vi "ParseDeviceData.vi"(8 "error in (no error)":errorcluster, 10 "Packet0":u8[](array[numeric])) -> (0 "error out":errorcluster, 2 "DataGood?":bool, 3 "Cluster":T1 {"DevInfo"."ASICtrim" format="%02x"})   [LabVIEW 2015]
uses:
  Controls/DeviceInfo.ctl
  Controls/InfoPacket.ctl
  Controls/Gen2 FT Globals.vi
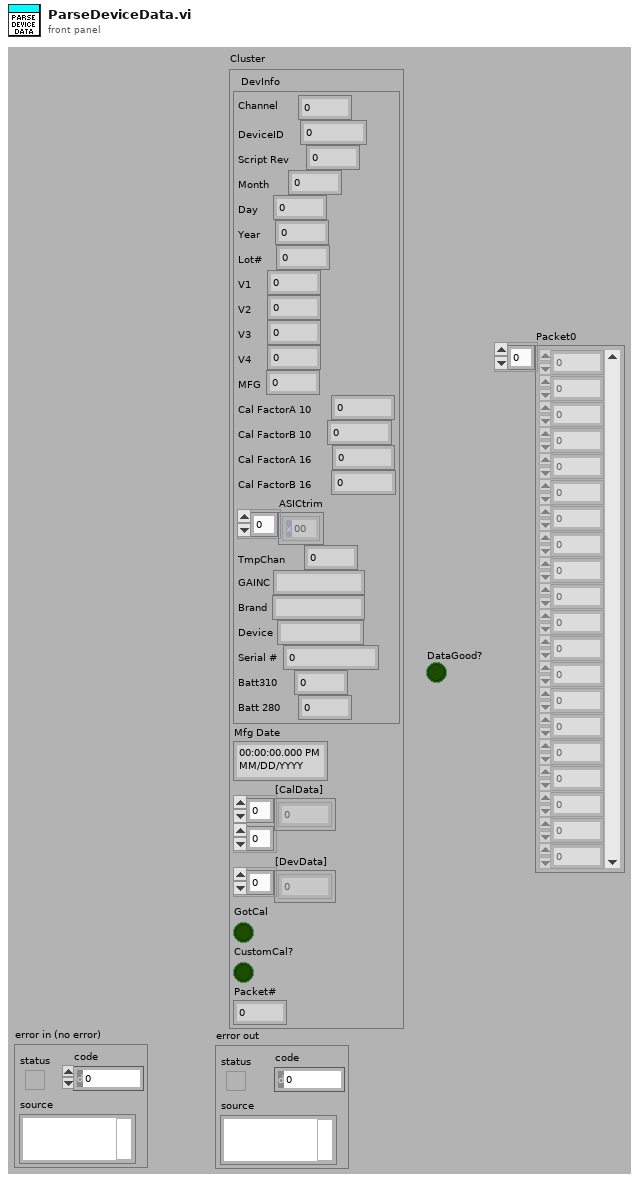
[diagram p1: front panel]
types:
  T1 = typedef "DeviceInfo.ctl" = cluster{"DevInfo":T2, "Mfg Date":timestamp, "[CalData]":u8[][], "[DevData]":u8[], "GotCal":bool, "CustomCal?":bool, "Packet#":i32}
  T2 = typedef "InfoPacket.ctl" = cluster{"Channel":u8, "DeviceID":u32, "Script Rev":u8, "Month":u8, "Day":u8, "Year":u8, "Lot#":u32, "V1":u16, "V2":u16, "V3":u16, "V4":u16, "MFG":u8, "Cal FactorA 10":u8, "Cal FactorB 10  ":u8, "Cal FactorA 16":u8, "Cal FactorB 16":u8, "ASICtrim":u8[], "TmpChan":u8, "GAINC":string, "Brand":string, "Device":string, "Serial #":u64, "Batt310":u16, "Batt 280":u16}
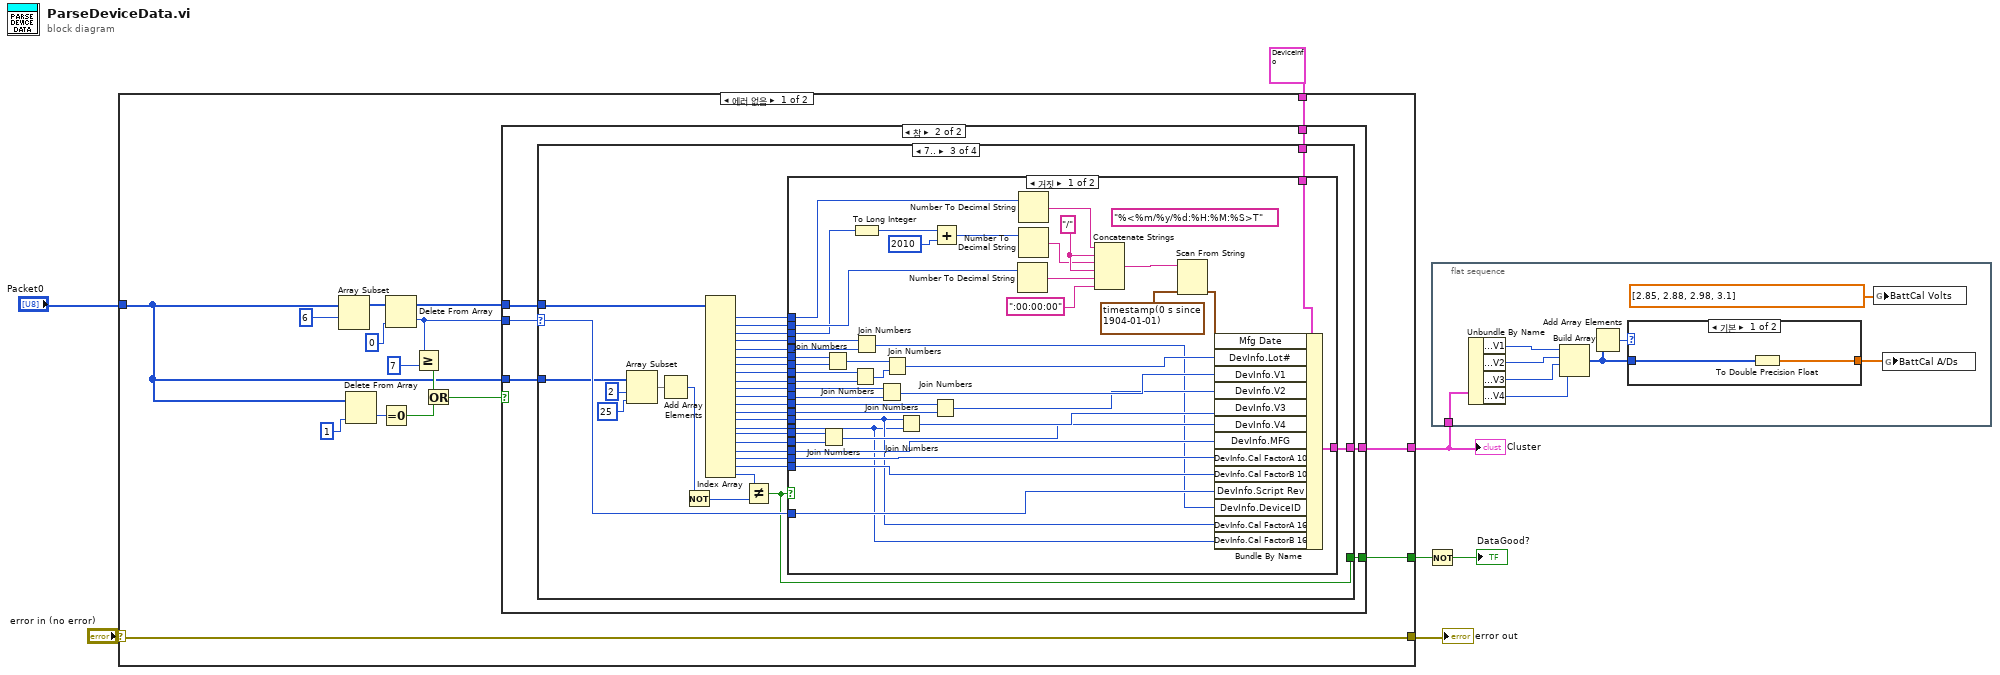
[diagram p0: block diagram]
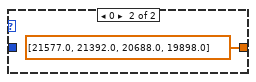
[diagram p2: hidden frame]
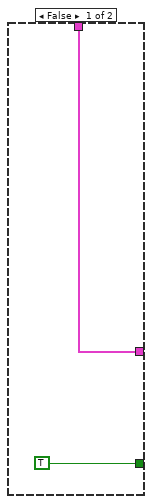
[diagram p3: hidden frame]
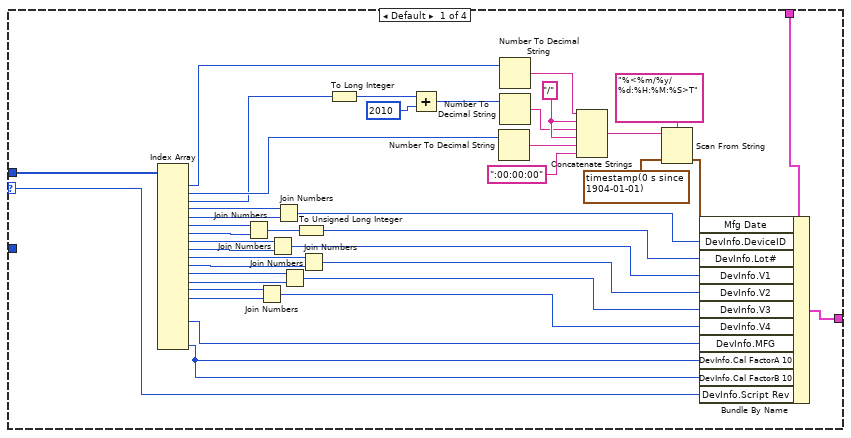
[diagram p4: hidden frame]
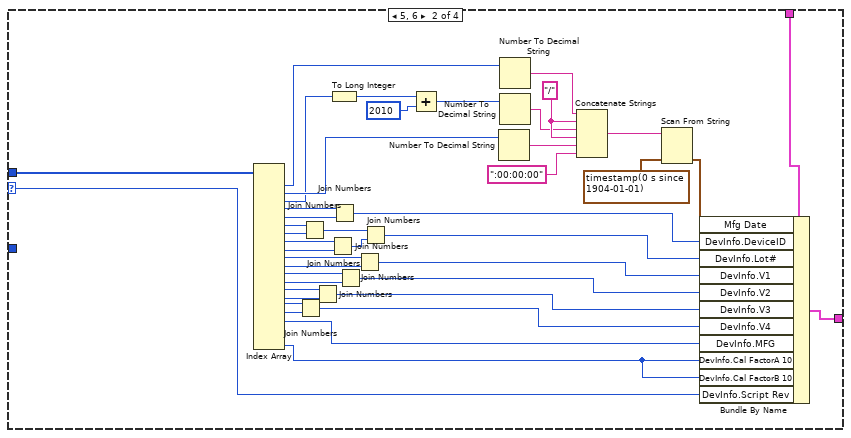
[diagram p5: hidden frame]
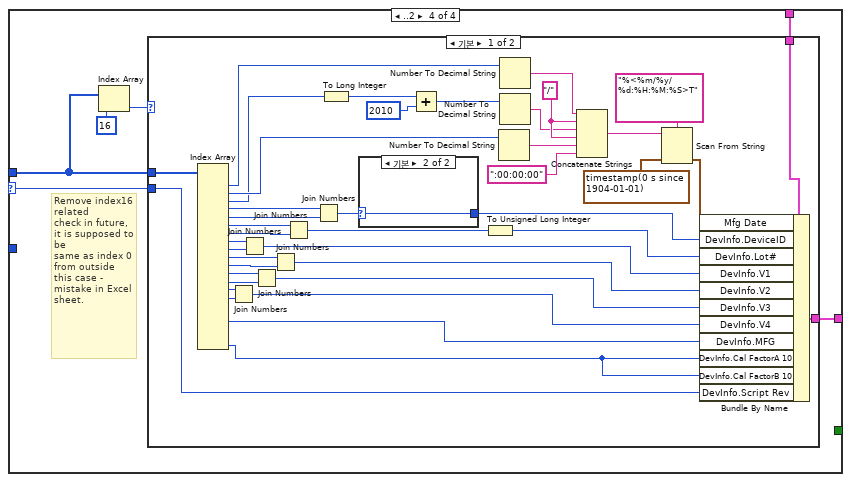
[diagram p7: hidden frame]
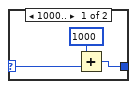
[diagram p8: hidden frame]
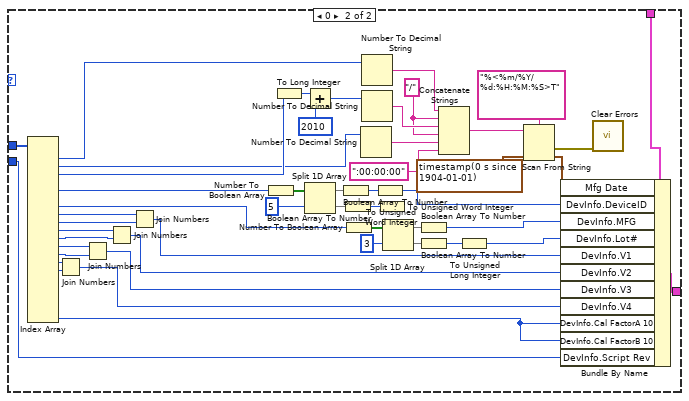
[diagram p9: hidden frame]
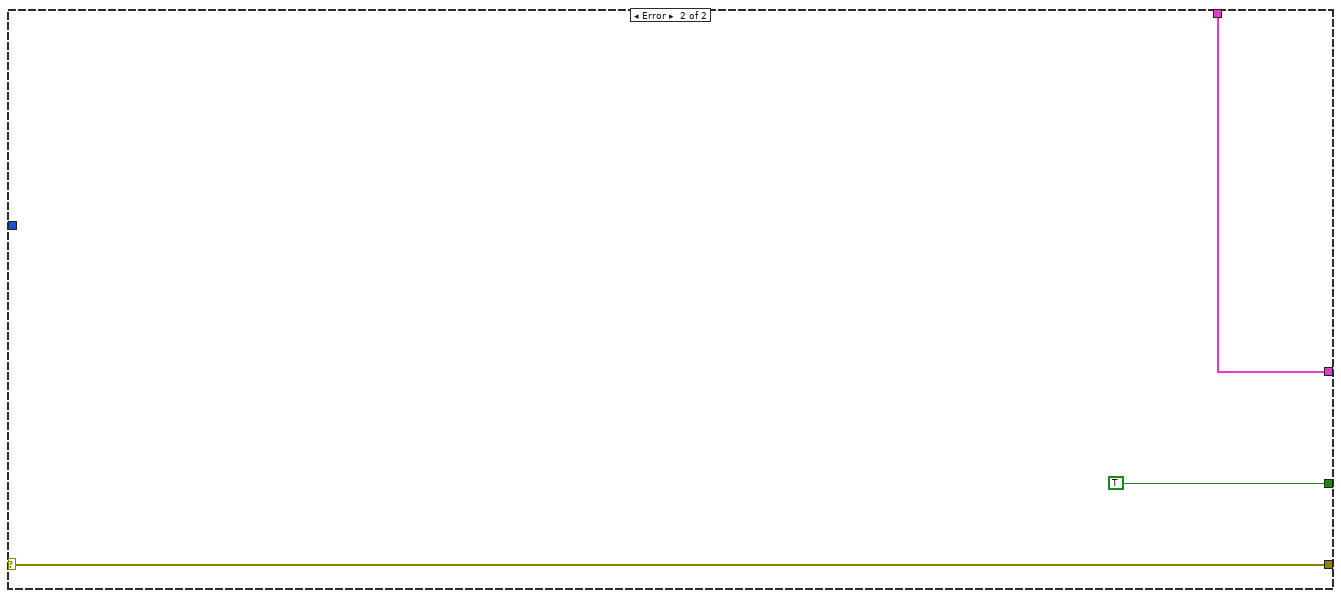
[diagram p10: hidden frame]
diagram:
  n1 = case shown="에러 없음" "error in (no error)" {
    selector: "error in (no error)" -> [w23 w291]
    tunnel: [w23 w291] -> w6
    tunnel: T1 {"DevInfo"={"Channel"=0, "DeviceID"=0, "Script Rev"=0, "Month"=0, "Day"=0, "Year"=0, "Lot#"=0, "V1"=0, "V2"=0, "V3"=0, "V4"=0, "MFG"=0, "Cal FactorA 10"=0, "Cal FactorB 10  "=0, "Cal FactorA 16"=0, "Cal FactorB 16"=0, "ASICtrim"=[], "TmpChan"=0, "GAINC"="", "Brand"="", "Device"="", "Serial #"=0, "Batt310"=0, "Batt 280"=0}, "Mfg Date"=timestamp(0 s since 1904-01-01), "[CalData]"=[], "[DevData]"=[], "GotCal"=FALSE, "CustomCal?"=FALSE, "Packet#"=0} -> [w22 w290]
    tunnel: [w21 w290] -> w3
    tunnel: "Packet0" -> [w8 _]
    tunnel: [w16 TRUE] -> w2
    frame No Error {
      n2 = Array Subset(array=w8, index=6) -> (w20:u8[])  [unwired: 1 in]
      n3 = Delete From Array(array=w8, index=1) -> (deleted portion=w14:u8)  [unwired: 1 in, 1 out]
      n4 = Equal To 0?(x=w14) -> (x = 0?=w9:bool)
      n5 = Delete From Array(array=w20, index=0) -> (deleted portion=w13:u8, array with subset deleted=w17:u8[])  [unwired: 1 in]
      n6 = Greater Or Equal?(x=w13, y=u8 7) -> (x >= y?=w10:bool)
      n7 = Or(x=w10, y=w9) -> (x .or. y?=w11:bool)
      n8 = case shown="참" w11 {
        tunnel: w22 -> [w25 w31]
        tunnel: [w25 w30] -> w21
        tunnel: w17 -> [_ w29]
        tunnel: w13 -> [_ w28]
        tunnel: [TRUE w27] -> w16
        tunnel: w8 -> [_ w26]
        frame False {
        }
        frame True {
          n9 = case shown="7.." w28 {
            selector: w28 -> [w68 w110 w143 w192]
            tunnel: w31 -> [w70 w112 w145 w194]
            tunnel: [w69 w111 w144 w193] -> w30
            tunnel: w29 -> [w71 w113 w122 w190]
            tunnel: w26 -> [_ _ w121 _]
            tunnel: [_ _ w114 _] -> w27
            frame Default {
              w58 = "/" ("string")
              n10 = Index Array(array=w71) -> (element #1=w63:u8, element #2=w64:u8, element #3=w52:u8, element #4=w66:u8, element #5=w67:u8, element #6=w50:u8, element #7=w51:u8, element #8=w47:u8, element #9=w46:u8, element #10=w45:u8, element #11=w44:u8, element #12=w43:u8, element #13=w42:u8, element #14=w41:u8, element #15=w40:u8, element #18=w38:u8, element #21=w32:u8)  [unwired: 21 in, 4 out]
              n11 = Join Numbers(hi=w50, lo=w51) -> ((hi.lo)=w39:u16)
              n12 = Join Numbers(hi=w41, lo=w40) -> ((hi.lo)=w33:u16)
              n13 = Join Numbers(hi=w47, lo=w46) -> ((hi.lo)=w36:u16)
              n14 = Join Numbers(hi=w66, lo=w67) -> ((hi.lo)=w48:u16)
              n15 = Join Numbers(hi=w43, lo=w42) -> ((hi.lo)=w34:u16)
              n16 = To Unsigned Long Integer(number=w39) -> (unsigned 32bit integer=w37:u32)
              n17 = Join Numbers(hi=w45, lo=w44) -> ((hi.lo)=w35:u16)
              n18 = To Long Integer(number=w52) -> (32bit integer=w54:i32)
              n19 = Add(x=w54, y=2010) -> (x+y=w65:i32)
              n20 = Number To Decimal String(number=w64) -> (decimal integer string=w59:string)  [unwired: 1 in]
              n21 = Number To Decimal String(number=w63) -> (decimal integer string=w56:string)  [unwired: 1 in]
              n22 = Number To Decimal String(number=w65) -> (decimal integer string=w57:string)  [unwired: 1 in]
              n23 = Concatenate Strings(w56, w58, w57, w58, w59, ":00:00:00" ("string")) -> (w62:string)
              n24 = Scan From String(format string="%<%m/%y/%d:%H:%M:%S>T", input string=w62, default 1=timestamp(0 s since 1904-01-01) ("current time")) -> (output 1=w49:timestamp)  [unwired: 2 in, 3 out]
              n25 = Bundle By Name(cluster=w70, "Mfg Date"=w49, "DevInfo.DeviceID"=w48, "DevInfo.Lot#"=w37, "DevInfo.V1"=w36, "DevInfo.V2"=w35, "DevInfo.V3"=w34, "DevInfo.V4"=w33, "DevInfo.MFG"=w38, "DevInfo.Cal FactorA 10"=w32, "DevInfo.Cal FactorB 10"=w32, "DevInfo.Script Rev"=w68) -> (w69:T1)
            }
            frame 5, 6 {
              w100 = "/" ("string")
              n26 = Index Array(array=w113) -> (element #1=w105:u8, element #2=w106:u8, element #3=w95:u8, element #4=w108:u8, element #5=w109:u8, element #6=w93:u8, element #7=w94:u8, element #8=w90:u8, element #9=w89:u8, element #10=w88:u8, element #11=w87:u8, element #12=w86:u8, element #13=w85:u8, element #14=w84:u8, element #15=w83:u8, element #16=w78:u8, element #17=w77:u8, element #18=w79:u8, element #21=w72:u8)  [unwired: 21 in, 2 out]
              n27 = Join Numbers(hi=w78, lo=w77) -> ((hi.lo)=w73:u16)
              n28 = Join Numbers(hi=w93, lo=w94) -> ((hi.lo)=w81:u16)
              n29 = Join Numbers(hi=w84, lo=w83) -> ((hi.lo)=w74:u16)
              n30 = Join Numbers(hi=w90, lo=w89) -> ((hi.lo)=w82:u16)
              n31 = To Long Integer(number=w95) -> (32bit integer=w97:i32)
              n32 = Join Numbers(hi=w108, lo=w109) -> ((hi.lo)=w91:u16)
              n33 = Join Numbers(hi=w86, lo=w85) -> ((hi.lo)=w75:u16)
              n34 = Join Numbers(hi=w88, lo=w87) -> ((hi.lo)=w76:u16)
              n35 = Join Numbers(hi=w81, lo=w82) -> ((hi.lo)=w80:u32)
              n36 = Add(x=w97, y=2010) -> (x+y=w107:i32)
              n37 = Number To Decimal String(number=w106) -> (decimal integer string=w101:string)  [unwired: 1 in]
              n38 = Number To Decimal String(number=w105) -> (decimal integer string=w98:string)  [unwired: 1 in]
              n39 = Number To Decimal String(number=w107) -> (decimal integer string=w99:string)  [unwired: 1 in]
              n40 = Concatenate Strings(w98, w100, w99, w100, w101, ":00:00:00" ("string")) -> (w104:string)
              n41 = Scan From String(input string=w104, default 1=timestamp(0 s since 1904-01-01) ("current time")) -> (output 1=w92:timestamp)  [unwired: 3 in, 3 out]
              n42 = Bundle By Name(cluster=w112, "Mfg Date"=w92, "DevInfo.DeviceID"=w91, "DevInfo.Lot#"=w80, "DevInfo.V1"=w76, "DevInfo.V2"=w75, "DevInfo.V3"=w74, "DevInfo.V4"=w73, "DevInfo.MFG"=w79, "DevInfo.Cal FactorA 10"=w72, "DevInfo.Cal FactorB 10"=w72, "DevInfo.Script Rev"=w110) -> (w111:T1)
            }
            frame 7.. {
              n43 = Array Subset(array=w121, index=2, length=25) -> (w118:u8[])
              n44 = Add Array Elements(numeric array=w118) -> (sum=w117:u8)
              n45 = Not(x=w117) -> (.not. x?=w115:u8)
              n46 = Index Array(array=w122) -> (element #1=w139:u8, element #2=w140:u8, element #3=w138:u8, element #4=w141:u8, element #5=w142:u8, element #6=w136:u8, element #7=w137:u8, element #8=w135:u8, element #9=w134:u8, element #10=w133:u8, element #11=w132:u8, element #12=w131:u8, element #13=w130:u8, element #14=w129:u8, element #15=w128:u8, element #16=w126:u8, element #17=w125:u8, element #18=w127:u8, element #19=w124:u8, element #20=w123:u8, element #21=w116:u8)  [unwired: 21 in]
              n47 = Not Equal?(x=w116, y=w115) -> (x != y?=w114:bool)
              n48 = case shown="거짓" w114 {
                tunnel: w145 -> [w187 w188]
                tunnel: [w186 w188] -> w144
                tunnel: w143 -> [w185 _]
                tunnel: w142 -> [w184 _]
                tunnel: w141 -> [w183 _]
                tunnel: w140 -> [w181 _]
                tunnel: w139 -> [w180 _]
                tunnel: w138 -> [w171 _]
                tunnel: w137 -> [w170 _]
                tunnel: w136 -> [w169 _]
                tunnel: w135 -> [w168 _]
                tunnel: w134 -> [w167 _]
                tunnel: w133 -> [w166 _]
                tunnel: w132 -> [w165 _]
                tunnel: w131 -> [w149 _]
                tunnel: w130 -> [w148 _]
                tunnel: w129 -> [w147 _]
                tunnel: w128 -> [w146 _]
                tunnel: w127 -> [w161 _]
                tunnel: w126 -> [w160 _]
                tunnel: w125 -> [w159 _]
                tunnel: w124 -> [w154 _]
                tunnel: w123 -> [w153 _]
                frame False {
                  (unwired) "%<%m/%y/%d:%H:%M:%S>T" ("format string")
                  w176 = "/" ("string")
                  n49 = Join Numbers(hi=w160, lo=w159) -> ((hi.lo)=w155:u16)
                  n50 = Join Numbers(hi=w169, lo=w170) -> ((hi.lo)=w163:u16)
                  n51 = Join Numbers(hi=w168, lo=w167) -> ((hi.lo)=w164:u16)
                  n52 = To Long Integer(number=w171) -> (32bit integer=w173:i32)
                  n53 = Join Numbers(hi=w183, lo=w184) -> ((hi.lo)=w152:u16)
                  n54 = Join Numbers(hi=w166, lo=w165) -> ((hi.lo)=w158:u16)
                  n55 = Join Numbers(hi=w163, lo=w164) -> ((hi.lo)=w162:u32)
                  n56 = Join Numbers(hi=w147, lo=w146) -> ((hi.lo)=w156:u16)
                  n57 = Join Numbers(hi=w149, lo=w148) -> ((hi.lo)=w157:u16)
                  n58 = Add(x=w173, y=2010) -> (x+y=w182:i32)
                  n59 = Number To Decimal String(number=w181) -> (decimal integer string=w177:string)  [unwired: 1 in]
                  n60 = Number To Decimal String(number=w180) -> (decimal integer string=w174:string)  [unwired: 1 in]
                  n61 = Number To Decimal String(number=w182) -> (decimal integer string=w175:string)  [unwired: 1 in]
                  n62 = Concatenate Strings(w174, w176, w175, w176, w177, ":00:00:00" ("string")) -> (w179:string)
                  n63 = Scan From String(input string=w179, default 1=timestamp(0 s since 1904-01-01) ("current time")) -> (output 1=w151:timestamp)  [unwired: 3 in, 3 out]
                  n64 = Bundle By Name(cluster=w187, "Mfg Date"=w151, "DevInfo.Lot#"=w162, "DevInfo.V1"=w158, "DevInfo.V2"=w157, "DevInfo.V3"=w156, "DevInfo.V4"=w155, "DevInfo.MFG"=w161, "DevInfo.Cal FactorA 10"=w154, "DevInfo.Cal FactorB 10"=w153, "DevInfo.Script Rev"=w185, "DevInfo.DeviceID"=w152, "DevInfo.Cal FactorA 16"=w147, "DevInfo.Cal FactorB 16"=w146) -> (w186:T1)
                }
                frame True {
                }
              }
            }
            frame ..2 {
              # "Remove index16 related\ncheck in future,\nit is supposed to be\nsame as index 0 from outside this case - mistake in Excel sheet."
              n65 = Index Array(array=w190, index=16) -> (element=w189:u8)
              n66 = case shown="기본" w189 {
                tunnel: w194 -> [w204 w288]
                tunnel: [w203 w287] -> w193
                tunnel: w190 -> [w235 w270]
                tunnel: w192 -> [w234 w258]
                frame Default {
                  w224 = "/" ("string")
                  n67 = Index Array(array=w235) -> (element #1=w229:u8, element #2=w230:u8, element #3=w218:u8, element #4=w232:u8, element #5=w233:u8, element #6=w216:u8, element #7=w217:u8, element #8=w214:u8, element #9=w213:u8, element #10=w212:u8, element #11=w211:u8, element #12=w210:u8, element #13=w209:u8, element #14=w208:u8, element #15=w207:u8, element #18=w205:u8, element #21=w195:u8)  [unwired: 21 in, 4 out]
                  n68 = Join Numbers(hi=w208, lo=w207) -> ((hi.lo)=w196:u16)
                  n69 = Join Numbers(hi=w214, lo=w213) -> ((hi.lo)=w199:u16)
                  n70 = Join Numbers(hi=w210, lo=w209) -> ((hi.lo)=w197:u16)
                  n71 = Join Numbers(hi=w212, lo=w211) -> ((hi.lo)=w198:u16)
                  n72 = Join Numbers(hi=w216, lo=w217) -> ((hi.lo)=w206:u16)
                  n73 = Join Numbers(hi=w232, lo=w233) -> ((hi.lo)=w202:u16)
                  n74 = To Long Integer(number=w218) -> (32bit integer=w220:i32)
                  n75 = case shown="기본" w202 {
                    selector: w202 -> [w238 w239]
                    tunnel: [w237 w239] -> w201
                    frame 1000.. {
                      n76 = Add(x=u16 1000, y=w238) -> (x+y=w237:u16)
                    }
                    frame Default {
                    }
                  }
                  n77 = Add(x=w220, y=2010) -> (x+y=w231:i32)
                  n78 = To Unsigned Long Integer(number=w206) -> (unsigned 32bit integer=w200:u32)
                  n79 = Number To Decimal String(number=w230) -> (decimal integer string=w225:string)  [unwired: 1 in]
                  n80 = Number To Decimal String(number=w229) -> (decimal integer string=w222:string)  [unwired: 1 in]
                  n81 = Number To Decimal String(number=w231) -> (decimal integer string=w223:string)  [unwired: 1 in]
                  n82 = Concatenate Strings(w222, w224, w223, w224, w225, ":00:00:00" ("string")) -> (w228:string)
                  n83 = Scan From String(format string="%<%m/%y/%d:%H:%M:%S>T", input string=w228, default 1=timestamp(0 s since 1904-01-01) ("current time")) -> (output 1=w215:timestamp)  [unwired: 2 in, 3 out]
                  n84 = Bundle By Name(cluster=w204, "Mfg Date"=w215, "DevInfo.DeviceID"=w201, "DevInfo.Lot#"=w200, "DevInfo.V1"=w199, "DevInfo.V2"=w198, "DevInfo.V3"=w197, "DevInfo.V4"=w196, "DevInfo.MFG"=w205, "DevInfo.Cal FactorA 10"=w195, "DevInfo.Cal FactorB 10"=w195, "DevInfo.Script Rev"=w234) -> (w203:T1)
                }
                frame 0 {
                  w278 = "/" ("string")
                  n85 = Index Array(array=w270) -> (element #1=w273:u8, element #2=w272:u8, element #3=w286:u8, element #5=w251:u8, element #7=w250:u8, element #8=w265:u8, element #9=w266:u8, element #10=w264:u8, element #11=w263:u8, element #12=w262:u8, element #13=w261:u8, element #14=w260:u8, element #15=w259:u8, element #21=w240:u8)  [unwired: 21 in, 7 out]
                  n86 = Join Numbers(hi=w260, lo=w259) -> ((hi.lo)=w241:u16)
                  n87 = Join Numbers(hi=w262, lo=w261) -> ((hi.lo)=w242:u16)
                  n88 = Join Numbers(hi=w264, lo=w263) -> ((hi.lo)=w243:u16)
                  n89 = Join Numbers(hi=w265, lo=w266) -> ((hi.lo)=w244:u16)
                  n90 = Number To Boolean Array(number=w251) -> (Boolean array=w283:bool[])
                  n91 = To Long Integer(number=w286) -> (32bit integer=w284:i32)
                  n92 = Add(x=w284, y=2010) -> (x+y=w271:i32)
                  n93 = Split 1D Array(array=w283, index=5) -> (first subarray=w257:bool[], second subarray=w245:bool[])
                  n94 = Boolean Array To Number(Boolean array=w257) -> (number=w256:u8)
                  n95 = Boolean Array To Number(Boolean array=w245) -> (number=w246:u8)
                  n96 = Number To Boolean Array(number=w250) -> (Boolean array=w255:bool[])
                  n97 = Number To Decimal String(number=w272) -> (decimal integer string=w277:string)  [unwired: 1 in]
                  n98 = Number To Decimal String(number=w273) -> (decimal integer string=w280:string)  [unwired: 1 in]
                  n99 = Number To Decimal String(number=w271) -> (decimal integer string=w279:string)  [unwired: 1 in]
                  n100 = To Unsigned Word Integer(number=w256) -> (unsigned 16bit integer=w268:u16)
                  n101 = To Unsigned Word Integer(number=w246) -> ()  [unwired: 1 out]
                  n102 = Split 1D Array(array=w255, index=3) -> (first subarray=w253:bool[], second subarray=w252:bool[])
                  n103 = Boolean Array To Number(Boolean array=w253) -> (number=w249:u8)
                  n104 = Boolean Array To Number(Boolean array=w252) -> (number=w248:u8)
                  n105 = Concatenate Strings(w280, w278, w279, w278, w277, ":00:00:00" ("string")) -> (w274:string)
                  n106 = To Unsigned Long Integer(number=w248) -> (unsigned 32bit integer=w247:u32)
                  n107 = Scan From String(format string="%<%m/%Y/%d:%H:%M:%S>T", input string=w274, default 1=timestamp(0 s since 1904-01-01) ("current time")) -> (error out=w269:errorcluster, output 1=w267:timestamp)  [unwired: 2 in, 2 out]
                  n108 = Bundle By Name(cluster=w288, "Mfg Date"=w267, "DevInfo.DeviceID"=w268, "DevInfo.MFG"=w249, "DevInfo.Lot#"=w247, "DevInfo.V1"=w244, "DevInfo.V2"=w243, "DevInfo.V3"=w242, "DevInfo.V4"=w241, "DevInfo.Cal FactorA 10"=w240, "DevInfo.Cal FactorB 10"=w240, "DevInfo.Script Rev"=w258) -> (w287:T1)
                  n109 = call <vilib>:"Clear Errors.vi"("error in (no error)"=w269) -> ()  [unwired: 5 in, 2 out]
                }
              }
            }
          }
        }
      }
    }
    frame Error {
    }
  }
  "error out" <- w6
  "Cluster" <- w3
  n110 = Not(x=w2) -> (.not. x?=→"DataGood?":bool)
  n111 = flat-sequence {
    tunnel: w3 -> [w296]
    frame #0 {
      n112 = Unbundle By Name(w296) -> ("DevInfo.V1"=w295:u16, "DevInfo.V2"=w294:u16, "DevInfo.V3"=w293:u16, "DevInfo.V4"=w292:u16)
      n113 = Build Array(w295, w294, w293, w292) -> (w300:u16[])
      n114 = Add Array Elements(numeric array=w300) -> (sum=w298:u16)
      n115 = case shown="기본" w298 {
        tunnel: w300 -> [w302 _]
        tunnel: [w301 dbl[] [21577.0, 21392.0, 20688.0, 19898.0] ("BattCal A/Ds")] -> w299
        frame Default {
          n116 = To Double Precision Float(number=w302) -> (double precision float=w301:dbl[])
        }
        frame 0 {
        }
      }
      n117 = global write "Gen2 FT Globals.vi" "BattCal Volts"(dbl[] [2.85, 2.88, 2.98, 3.1] ("BattCal A/Ds")) -> ()
      n118 = global write "Gen2 FT Globals.vi" "BattCal A/Ds"(w299) -> ()
    }
  }
